vi "Analog IO.vi"() -> ()   [LabVIEW 2011]
panel:
  out "Ch9 Data 2":dbl
  out "Ch0 Data 2":dbl
  out "Ch1 Data 2":dbl
  out "Ch6 Data 2":dbl
  out "Ch2 Data 2":dbl
  out "Ch7 Data 2":dbl
  out "Ch10 Data 2":dbl
  out "Ch12 Data 2":dbl
  out "Ch13 Data 2":dbl
  out "Ch4 Data 2":dbl
  out "Ch3 Data 2":dbl
  out "Ch15 Data 2":dbl
  out "Ch14 Data 2":dbl
  out "Ch5 Data 2":dbl
  out "Ch8 Data 2":dbl
  out "Ch11 Data 2":dbl
  in  "Ch9 Range Type":i16
  in  "Ch0 Range Type":i16
  in  "Ch1 Range Type":i16
  in  "Ch6 Range Type":i16
  in  "Ch2 Range Type":i16
  in  "Ch7 Range Type":i16
  in  "Ch10 Range Type":i16
  in  "Ch12 Range Type":i16
  in  "Ch13 Range Type":i16
  in  "Ch4 Range Type":i16
  in  "Ch3 Range Type":i16
  in  "Ch15 Range Type":i16
  in  "Ch14 Range Type":i16
  in  "Ch5 Range Type":i16
  in  "Ch8 Range Type":i16
  in  "Ch11 Range Type":i16
  in  "Ch0 Data":i16
  in  "Ch15 Data":i16
  in  "Ch14 Data":i16
  in  "Ch13 Data":i16
  in  "Ch12 Data":i16
  in  "Ch11 Data":i16
  in  "Ch10 Data":i16
  in  "Ch9 Data":i16
  in  "Ch8 Data":i16
  in  "Ch7 Data":i16
  in  "Ch6 Data":i16
  in  "Ch5 Data":i16
  in  "Ch4 Data":i16
  in  "Ch3 Data":i16
  in  "Ch2 Data":i16
  in  "Ch1 Data":i16
  out "CalFault":bool
  out "Calibrating":bool
  out "AnalogGroupFault":bool
  in  "Channel Status":u32 format="%032b"
  out "Ch1Underrange":bool
  out "Ch15Underrange":bool
  out "Ch14Underrange":bool
  out "Ch13Underrange":bool
  out "Ch12Underrange":bool
  out "Ch11Underrange":bool
  out "Ch10Underrange":bool
  out "Ch9Underrange":bool
  out "Ch8Underrange":bool
  out "Ch7Underrange":bool
  out "Ch6Underrange":bool
  out "Ch5Underrange":bool
  out "Ch4Underrange":bool
  out "Ch3Underrange":bool
  out "Ch2Underrange":bool
  out "Ch0Underrange":bool
  out "Ch1Overrange":bool
  out "Ch15Overrange":bool
  out "Ch14Overrange":bool
  out "Ch13Overrange":bool
  out "Ch12Overrange":bool
  out "Ch11Overrange":bool
  out "Ch10Overrange":bool
  out "Ch9Overrange":bool
  out "Ch8Overrange":bool
  out "Ch7Overrange":bool
  out "Ch6Overrange":bool
  out "Ch5Overrange":bool
  out "Ch4Overrange":bool
  out "Ch3Overrange":bool
  out "Ch2Overrange":bool
  out "Ch0Overrange":bool
  out "Module 1":bool
  out "Module 12":bool
  out "Module 15":bool
  out "Module 14":bool
  out "Module 13":bool
  out "Module 11":bool
  out "Module 10":bool
  out "Module 9":bool
  out "Module 8":bool
  out "Module 7":bool
  out "Module 6":bool
  out "Module 5":bool
  out "Module 4":bool
  out "Module 3":bool
  out "Module 2":bool
  out "Module 0":bool
  in  "Module Faults":u16 format="%016b"
  out "Channel 1":bool
  out "Channel 15":bool
  out "Channel 14":bool
  out "Channel 13":bool
  out "Channel 12":bool
  out "Channel 11":bool
  out "Channel 10":bool
  out "Channel 9":bool
  out "Channel 8":bool
  out "Channel 7":bool
  out "Channel 6":bool
  out "Channel 5":bool
  out "Channel 4":bool
  out "Channel 3":bool
  out "Channel 2":bool
  out "Channel 0":bool
  in  "Analog Module":bool
  in  "URL":string="opc://localhost/National Instruments.NIOPCServers/ABOPC.ABEthernet.Global"
  in  "Stop Button":bool
  in  "Channel Faults":u16 format="%016b"
  # "(Volts)"
  # "Channel\nRange\nType"
  # "Channel Ranges"
  # "Channel\nFaults"
  # "Module\nFaults"
  # "Channel\nData"
  # "Under"
  # "Over"
  # "CH 0"
  # "CH 1"
  # "CH 2"
  # "CH 3"
  # "CH 4"
  # "CH 5"
  # "CH 6"
  # "CH 7"
  # "CH 8"
  # "CH 9"
  # "CH 10"
  # "CH 11"
  # "CH 12"
  # "CH 13"
  # "CH 14"
  # "CH 15"
  # "5"
  # "6"
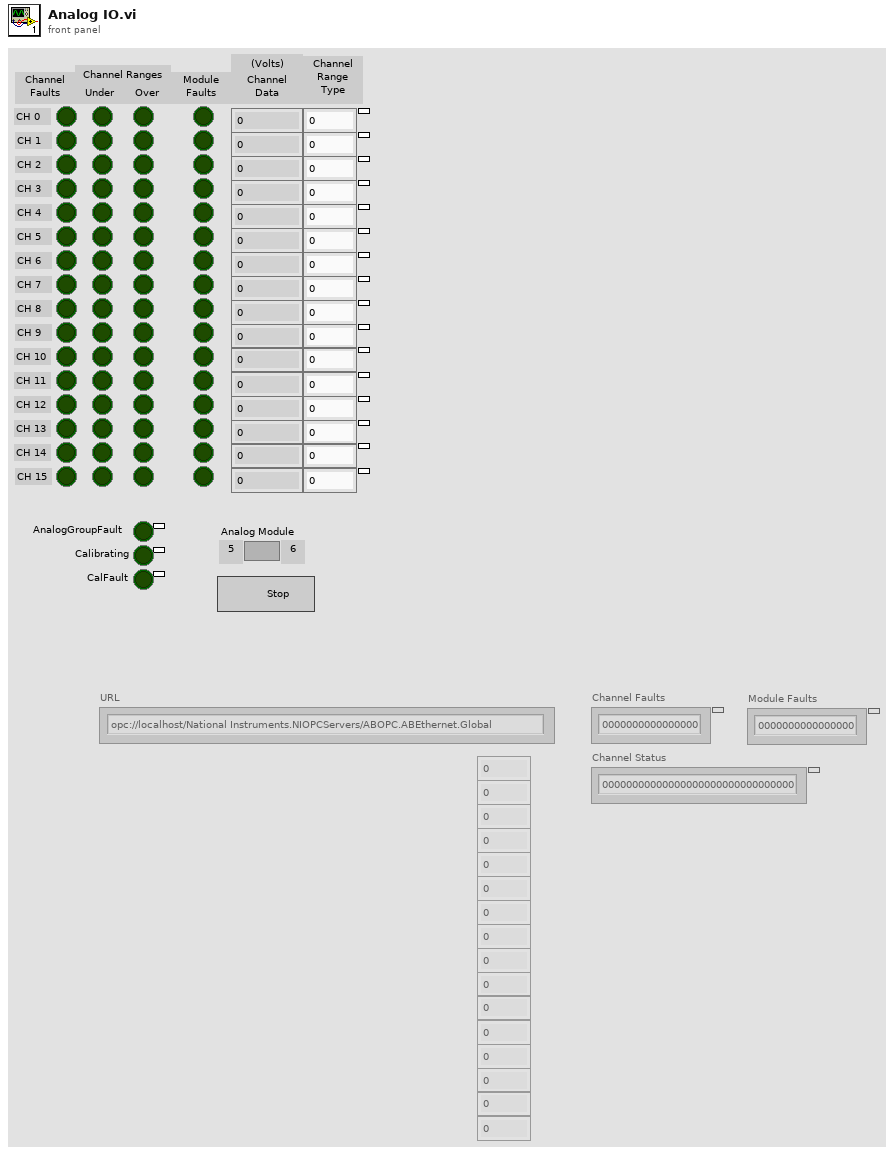
[diagram p1: front panel]
types:
  T1 = cluster{"Boolean array[0]":bool, "Boolean array[1]":bool, "Boolean array[2]":bool, "Boolean array[3]":bool, "Boolean array[4]":bool, "Boolean array[5]":bool, "Boolean array[6]":bool, "Boolean array[7]":bool, "Boolean array[8]":bool, "Boolean array[9]":bool, "Boolean array[10]":bool, "Boolean array[11]":bool, "Boolean array[12]":bool, "Boolean array[13]":bool, "Boolean array[14]":bool, "Boolean array[15]":bool}
  T2 = cluster{"[0]":dbl, "[1]":dbl, "[2]":dbl, "[3]":dbl, "[4]":dbl, "[5]":dbl, "[6]":dbl, "[7]":dbl, "[8]":dbl, "[9]":dbl, "[10]":dbl, "[11]":dbl, "[12]":dbl, "[13]":dbl, "[14]":dbl, "[15]":dbl}
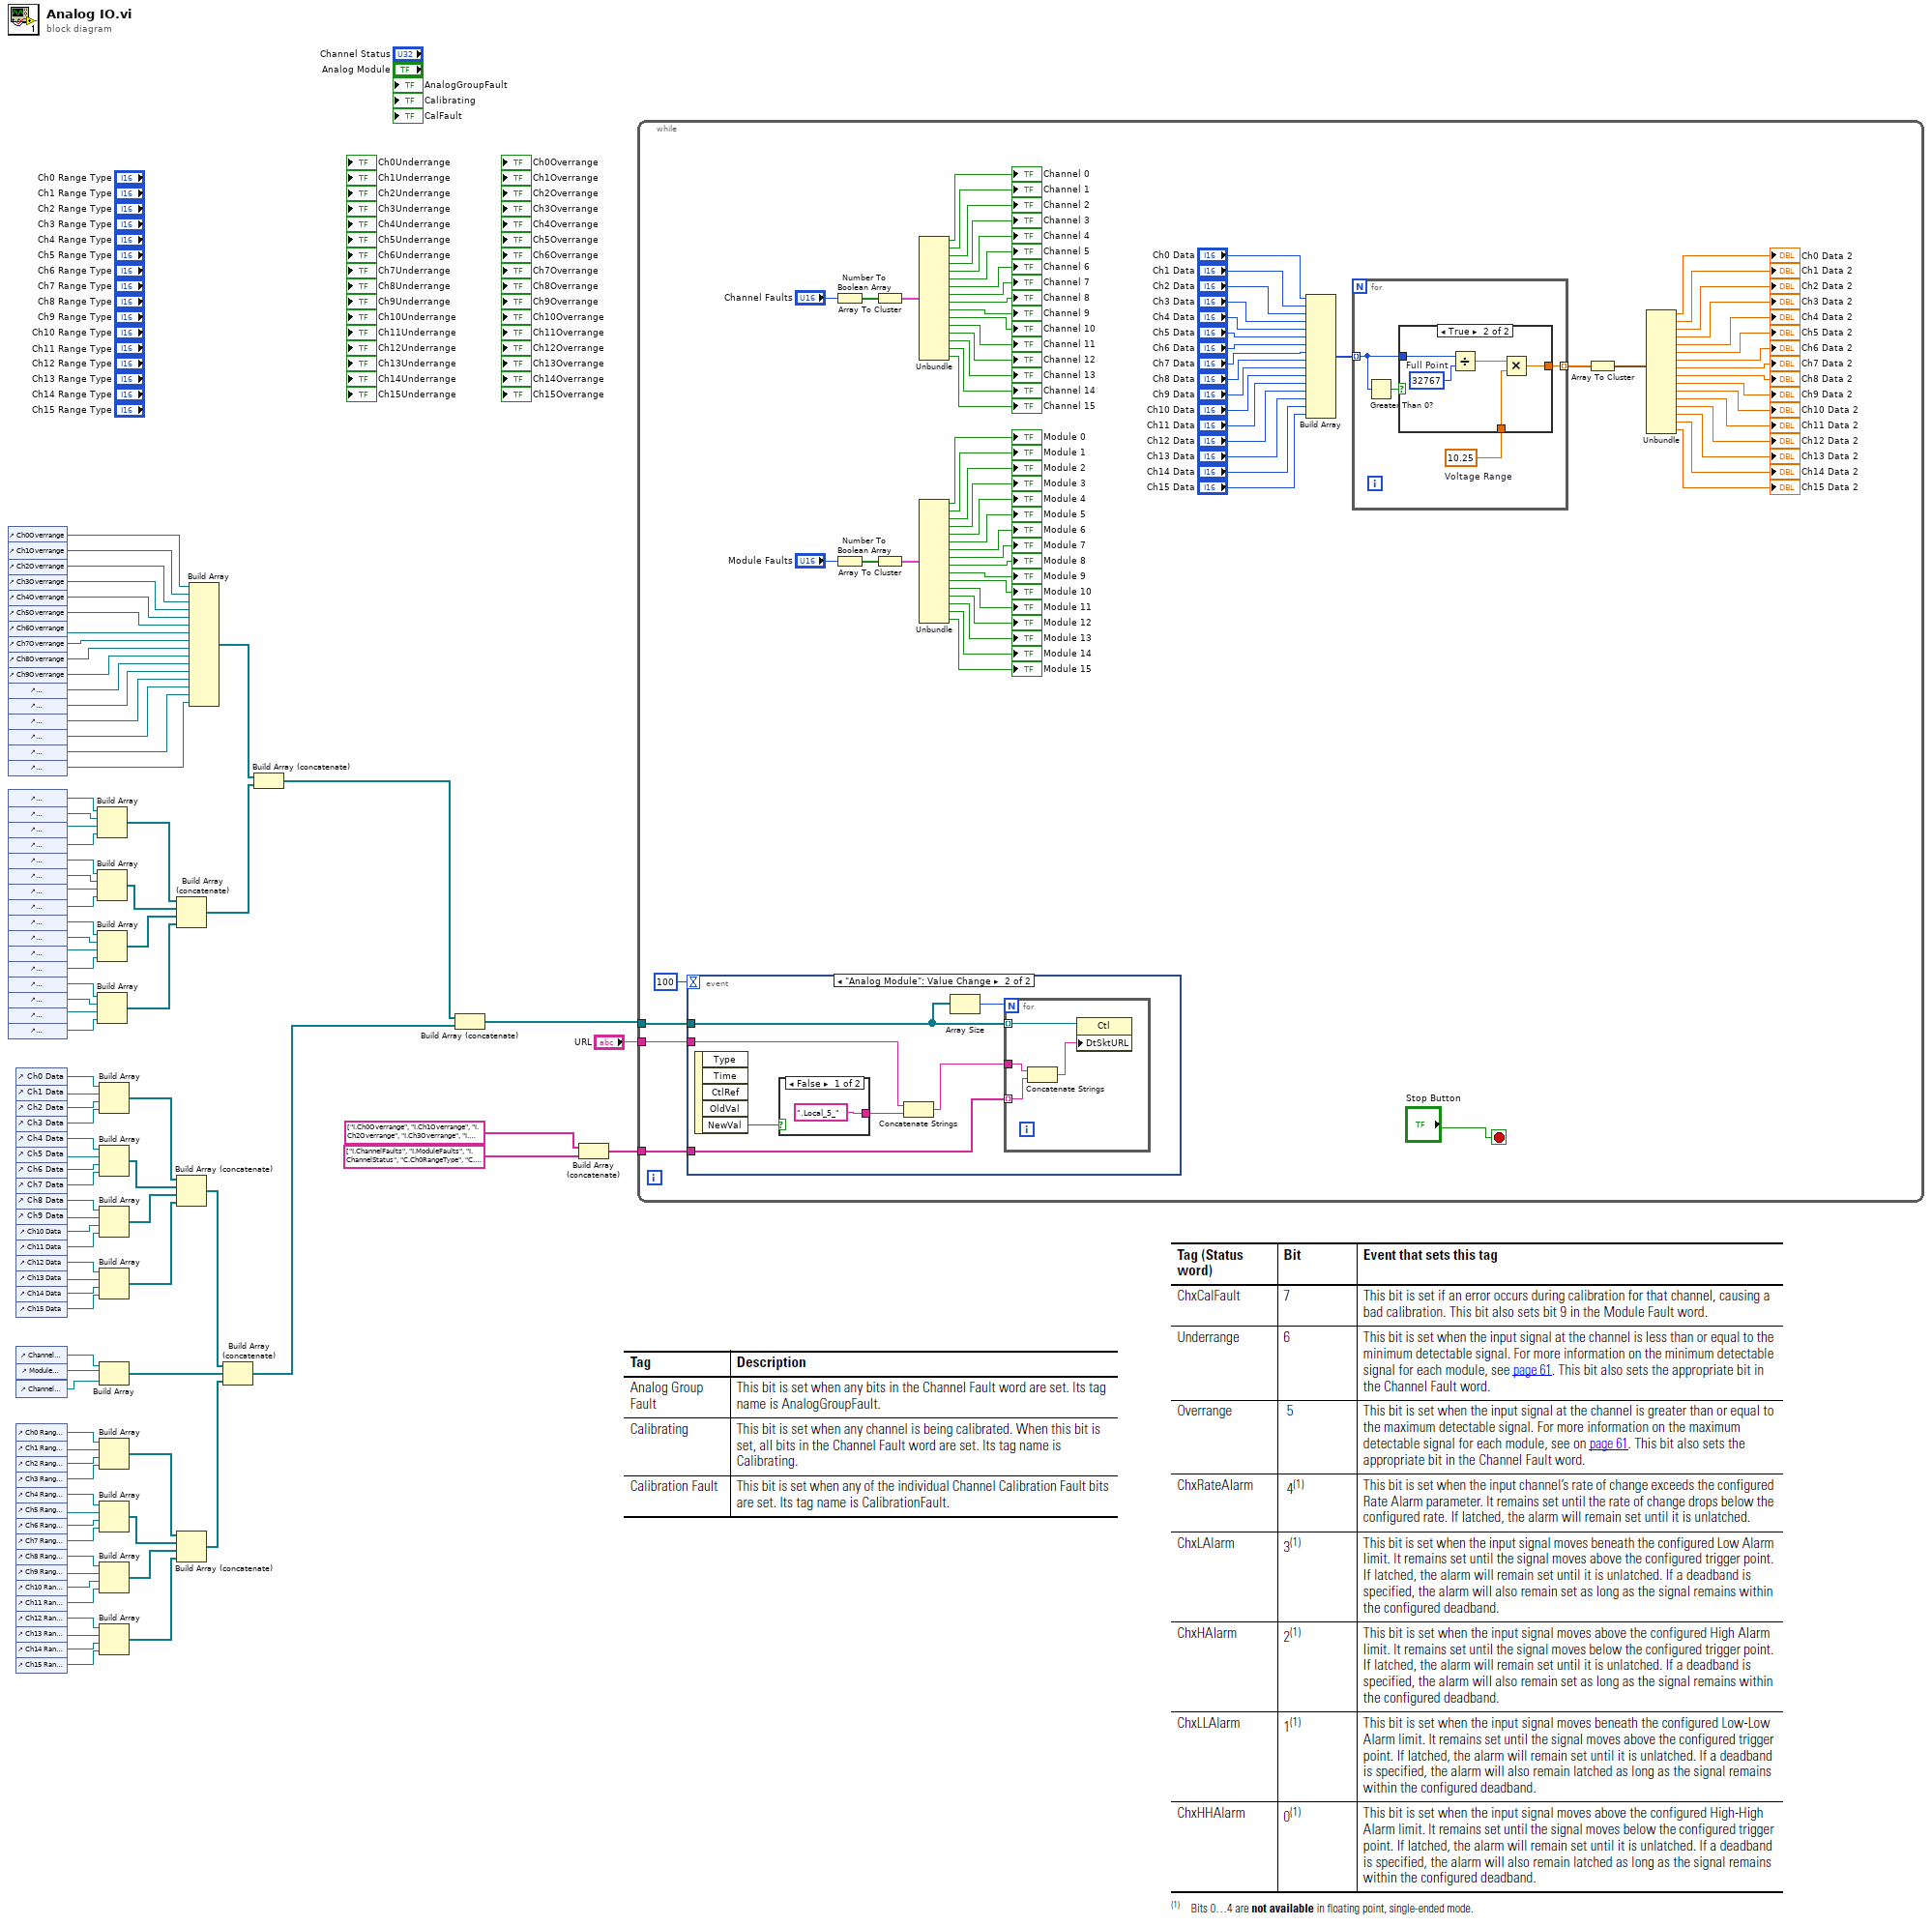
[diagram p0: block diagram]
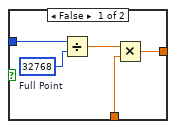
[diagram p2: hidden frame]
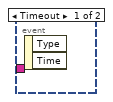
[diagram p3: hidden frame]
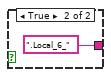
[diagram p4: hidden frame]
diagram:
  n1 = control-ref of="Ch0Overrange"() -> (w91:refnum<vi>)
  n2 = control-ref of="Ch1Overrange"() -> (w90:refnum<vi>)
  n3 = control-ref of="Ch2Overrange"() -> (w89:refnum<vi>)
  n4 = control-ref of="Ch3Overrange"() -> (w88:refnum<vi>)
  n5 = control-ref of="Ch4Overrange"() -> (w87:refnum<vi>)
  n6 = control-ref of="Ch5Overrange"() -> (w86:refnum<vi>)
  n7 = control-ref of="Ch6Overrange"() -> (w85:refnum<vi>)
  n8 = control-ref of="Ch7Overrange"() -> (w84:refnum<vi>)
  n9 = control-ref of="Ch8Overrange"() -> (w83:refnum<vi>)
  n10 = control-ref of="Ch9Overrange"() -> (w82:refnum<vi>)
  n11 = control-ref of="Ch10Overrange"() -> (w81:refnum<vi>)
  n12 = control-ref of="Ch11Overrange"() -> (w80:refnum<vi>)
  n13 = control-ref of="Ch12Overrange"() -> (w79:refnum<vi>)
  n14 = control-ref of="Ch13Overrange"() -> (w78:refnum<vi>)
  n15 = control-ref of="Ch14Overrange"() -> (w77:refnum<vi>)
  n16 = control-ref of="Ch15Overrange"() -> (w76:refnum<vi>)
  n17 = control-ref of="Ch0Underrange"() -> (w74:refnum<vi>)
  n18 = control-ref of="Ch1Underrange"() -> (w73:refnum<vi>)
  n19 = control-ref of="Ch2Underrange"() -> (w72:refnum<vi>)
  n20 = control-ref of="Ch3Underrange"() -> (w71:refnum<vi>)
  n21 = control-ref of="Ch4Underrange"() -> (w70:refnum<vi>)
  n22 = control-ref of="Ch5Underrange"() -> (w69:refnum<vi>)
  n23 = control-ref of="Ch6Underrange"() -> (w68:refnum<vi>)
  n24 = control-ref of="Ch7Underrange"() -> (w67:refnum<vi>)
  n25 = control-ref of="Ch8Underrange"() -> (w66:refnum<vi>)
  n26 = control-ref of="Ch9Underrange"() -> (w65:refnum<vi>)
  n27 = control-ref of="Ch10Underrange"() -> (w64:refnum<vi>)
  n28 = control-ref of="Ch11Underrange"() -> (w63:refnum<vi>)
  n29 = control-ref of="Ch12Underrange"() -> (w62:refnum<vi>)
  n30 = control-ref of="Ch13Underrange"() -> (w61:refnum<vi>)
  n31 = control-ref of="Ch14Underrange"() -> (w60:refnum<vi>)
  n32 = control-ref of="Ch15Underrange"() -> (w59:refnum<vi>)
  n33 = control-ref of="Ch0 Data"() -> (w50:refnum<vi>)
  n34 = control-ref of="Ch1 Data"() -> (w49:refnum<vi>)
  n35 = control-ref of="Ch2 Data"() -> (w48:refnum<vi>)
  n36 = control-ref of="Ch3 Data"() -> (w47:refnum<vi>)
  n37 = control-ref of="Ch4 Data"() -> (w46:refnum<vi>)
  n38 = control-ref of="Ch5 Data"() -> (w45:refnum<vi>)
  n39 = control-ref of="Ch6 Data"() -> (w44:refnum<vi>)
  n40 = control-ref of="Ch7 Data"() -> (w43:refnum<vi>)
  n41 = control-ref of="Ch8 Data"() -> (w42:refnum<vi>)
  n42 = control-ref of="Ch9 Data"() -> (w41:refnum<vi>)
  n43 = control-ref of="Ch10 Data"() -> (w39:refnum<vi>)
  n44 = control-ref of="Ch11 Data"() -> (w40:refnum<vi>)
  n45 = control-ref of="Ch12 Data"() -> (w38:refnum<vi>)
  n46 = control-ref of="Ch13 Data"() -> (w37:refnum<vi>)
  n47 = control-ref of="Ch14 Data"() -> (w36:refnum<vi>)
  n48 = control-ref of="Ch15 Data"() -> (w35:refnum<vi>)
  n49 = control-ref of="Channel Faults"() -> (w32:refnum<vi>)
  n50 = control-ref of="Module Faults"() -> (w33:refnum<vi>)
  n51 = control-ref of="Channel Status"() -> (w34:refnum<vi>)
  n52 = control-ref of="Ch0 Range Type"() -> (w19:refnum<vi>)
  n53 = control-ref of="Ch1 Range Type"() -> (w18:refnum<vi>)
  n54 = control-ref of="Ch2 Range Type"() -> (w17:refnum<vi>)
  n55 = control-ref of="Ch3 Range Type"() -> (w16:refnum<vi>)
  n56 = control-ref of="Ch4 Range Type"() -> (w15:refnum<vi>)
  n57 = control-ref of="Ch5 Range Type"() -> (w14:refnum<vi>)
  n58 = control-ref of="Ch6 Range Type"() -> (w13:refnum<vi>)
  n59 = control-ref of="Ch7 Range Type"() -> (w12:refnum<vi>)
  n60 = control-ref of="Ch8 Range Type"() -> (w11:refnum<vi>)
  n61 = control-ref of="Ch9 Range Type"() -> (w10:refnum<vi>)
  n62 = control-ref of="Ch10 Range Type"() -> (w8:refnum<vi>)
  n63 = control-ref of="Ch11 Range Type"() -> (w9:refnum<vi>)
  n64 = control-ref of="Ch12 Range Type"() -> (w7:refnum<vi>)
  n65 = control-ref of="Ch13 Range Type"() -> (w6:refnum<vi>)
  n66 = control-ref of="Ch14 Range Type"() -> (w5:refnum<vi>)
  n67 = control-ref of="Ch15 Range Type"() -> (w4:refnum<vi>)
  n68 = Build Array(w74, w73, w72, w71) -> (w58:refnum<vi>[])
  n69 = Build Array(w70, w69, w68, w67) -> (w57:refnum<vi>[])
  n70 = Build Array(w66, w65, w64, w63) -> (w56:refnum<vi>[])
  n71 = Build Array(w62, w61, w60, w59) -> (w55:refnum<vi>[])
  n72 = Build Array(w50, w49, w48, w47) -> (w54:refnum<vi>[])
  n73 = Build Array(w46, w45, w44, w43) -> (w53:refnum<vi>[])
  n74 = Build Array(w42, w41, w39, w40) -> (w52:refnum<vi>[])
  n75 = Build Array(w38, w37, w36, w35) -> (w51:refnum<vi>[])
  n76 = Build Array(w32, w33, w34) -> (w2:refnum<vi>[])
  n77 = Build Array(w19, w18, w17, w16) -> (w23:refnum<vi>[])
  n78 = Build Array(w15, w14, w13, w12) -> (w22:refnum<vi>[])
  n79 = Build Array(w11, w10, w8, w9) -> (w21:refnum<vi>[])
  n80 = Build Array(w7, w6, w5, w4) -> (w20:refnum<vi>[])
  n81 = Build Array (concatenate)(w58, w57, w56, w55) -> (w30:refnum<vi>[])
  n82 = Build Array (concatenate)(w54, w53, w52, w51) -> (w3:refnum<vi>[])
  n83 = Build Array (concatenate)(w23, w22, w21, w20) -> (w1:refnum<vi>[])
  n84 = Build Array(w91, w90, w89, w88, w87, w86, w85, w84, w83, w82, w81, w80, w79, w78, w77, w76) -> (w31:refnum<vi>[])
  n85 = Build Array (concatenate)(w3, w2, w1) -> (w27:refnum<vi>[])
  n86 = Build Array (concatenate)(w31, w30) -> (w28:refnum<vi>[])
  n87 = Build Array (concatenate)(w28, w27) -> (w29:refnum<vi>[])
  n88 = Build Array (concatenate)(string[] ["I.Ch0Overrange", "I.Ch1Overrange", "I.Ch2Overrange", "I.Ch3Overrange", "I.Ch4Overrange", "I.Ch5Overrange", "I.Ch6Overrange", "I.Ch7Overrange", "I.Ch8Overrange", "I.Ch9Overrange", "I.Ch10Overrange", "I.Ch11Overrange", "I.Ch12Overrange", "I.Ch13Overrange", "I.Ch14Overrange", "I.Ch15Overrange", "I.Ch0Underrange", "I.Ch1Underrange", "I.Ch2Underrange", "I.Ch3Underrange", "I.Ch4Underrange", "I.Ch5Underrange", "I.Ch6Underrange", "I.Ch7Underrange", "I.Ch8Underrange", "I.Ch9Underrange", "I.Ch10Underrange", "I.Ch11Underrange", "I.Ch12Underrange", "I.Ch13Underrange", "I.Ch14Underrange", "I.Ch15Underrange", "I.Ch0Data", "I.Ch1Data", "I.Ch2Data", "I.Ch3Data", "I.Ch4Data", "I.Ch5Data", "I.Ch6Data", "I.Ch7Data", "I.Ch8Data", "I.Ch9Data", "I.Ch10Data", "I.Ch11Data", "I.Ch12Data", "I.Ch13Data", "I.Ch14Data", "I.Ch15Data"], string[] ["I.ChannelFaults", "I.ModuleFaults", "I.ChannelStatus", "C.Ch0RangeType", "C.Ch1RangeType", "C.Ch2RangeType", "C.Ch3RangeType", "C.Ch4RangeType", "C.Ch5RangeType", "C.Ch6RangeType", "C.Ch7RangeType", "C.Ch8RangeType", "C.Ch9RangeType", "C.Ch10RangeType", "C.Ch11RangeType", "C.Ch12RangeType", "C.Ch13RangeType", "C.Ch14RangeType", "C.Ch15RangeType"]) -> (w24:string[])
  n89 = while {
    tunnel: "URL" -> [w167]
    tunnel: w24 -> [w128]
    tunnel: w29 -> [w127]
    stop <- "Stop Button" stop-if-true
    n90 = event shown="[1] \"Analog Module\": Value Change" {
      selector: _ -> [_ _]
      dyn-events: _ -> [_ _]
      timeout: 100 -> [_ _]
      tunnel: w167 -> [_ w187]
      tunnel: w128 -> [_ w189]
      tunnel: w127 -> [_ w184]
      event Timeout {
        n91 = event-data() -> ()  [unwired: 1 in, 2 out]
      }
      event "Analog Module": Value Change {
        n92 = event-data() -> ("NewVal"=w190:bool)  [unwired: 1 in, 4 out]
        n93 = case shown="False" w190 {
          tunnel: [".Local_5_" ".Local_6_"] -> w188
          frame False {
          }
          frame True {
          }
        }
        n94 = Concatenate Strings(w187, w188) -> (w186:string)
        n95 = Array Size(array=w184) -> (size(s)=w185:i32)
        n96 = for {
          N: w185 -> [_]
          tunnel: w189 -> [w194] mode=indexing
          tunnel: w184 -> [w191] mode=indexing
          tunnel: w186 -> [w192]
          n97 = Concatenate Strings(w192, w194) -> (w193:string)
          n98 = property on="Property Node" class="Ctl"(reference=w191, "DtSktURL"=w193) -> ()  [unwired: 1 in, 2 out]
        }
      }
    }
    n99 = Number To Boolean Array(number="Channel Faults") -> (Boolean array=w165:bool[])
    n100 = Number To Boolean Array(number="Module Faults") -> (Boolean array=w147:bool[])
    n101 = Array To Cluster(array=w165) -> (cluster=w164:T1)
    n102 = Array To Cluster(array=w147) -> (cluster=w146:T1)
    n103 = Unbundle(w164) -> ("Boolean array[0]"=→"Channel 0":bool, "Boolean array[1]"=→"Channel 1":bool, "Boolean array[2]"=→"Channel 2":bool, "Boolean array[3]"=→"Channel 3":bool, "Boolean array[4]"=→"Channel 4":bool, "Boolean array[5]"=→"Channel 5":bool, "Boolean array[6]"=→"Channel 6":bool, "Boolean array[7]"=→"Channel 7":bool, "Boolean array[8]"=→"Channel 8":bool, "Boolean array[9]"=→"Channel 9":bool, "Boolean array[10]"=→"Channel 10":bool, "Boolean array[11]"=→"Channel 11":bool, "Boolean array[12]"=→"Channel 12":bool, "Boolean array[13]"=→"Channel 13":bool, "Boolean array[14]"=→"Channel 14":bool, "Boolean array[15]"=→"Channel 15":bool)
    n104 = Unbundle(w146) -> ("Boolean array[0]"=→"Module 0":bool, "Boolean array[1]"=→"Module 1":bool, "Boolean array[2]"=→"Module 2":bool, "Boolean array[3]"=→"Module 3":bool, "Boolean array[4]"=→"Module 4":bool, "Boolean array[5]"=→"Module 5":bool, "Boolean array[6]"=→"Module 6":bool, "Boolean array[7]"=→"Module 7":bool, "Boolean array[8]"=→"Module 8":bool, "Boolean array[9]"=→"Module 9":bool, "Boolean array[10]"=→"Module 10":bool, "Boolean array[11]"=→"Module 11":bool, "Boolean array[12]"=→"Module 12":bool, "Boolean array[13]"=→"Module 13":bool, "Boolean array[14]"=→"Module 14":bool, "Boolean array[15]"=→"Module 15":bool)
    n105 = Build Array("Ch0 Data", "Ch1 Data", "Ch2 Data", "Ch3 Data", "Ch4 Data", "Ch5 Data", "Ch6 Data", "Ch7 Data", "Ch8 Data", "Ch9 Data", "Ch10 Data", "Ch11 Data", "Ch12 Data", "Ch13 Data", "Ch14 Data", "Ch15 Data") -> (w110:i16[])
    n106 = for {
      tunnel: w110 -> [w172] mode=indexing
      tunnel: [w173] -> w109 mode=indexing
      w170 = 10.25  # Voltage Range
      n107 = Greater Than 0?(x=w172) -> (x > 0?=w171:bool)
      n108 = case shown="True" w171 {
        tunnel: w172 -> [w175 w183]
        tunnel: [w174 w181] -> w173
        tunnel: w170 -> [w176 w180]
        frame False {
          w177 = 32768  # Full Point
          n109 = Divide(x=w175, y=w177) -> (x/y=w178:dbl)
          n110 = Multiply(x=w178, y=w176) -> (x*y=w174:dbl)
        }
        frame True {
          w179 = 32767  # Full Point
          n111 = Divide(x=w183, y=w179) -> (x/y=w182:dbl)
          n112 = Multiply(x=w182, y=w180) -> (x*y=w181:dbl)
        }
      }
    }
    n113 = Array To Cluster(array=w109) -> (cluster=w108:T2)
    n114 = Unbundle(w108) -> ("[0]"=→"Ch0 Data 2":dbl, "[1]"=→"Ch1 Data 2":dbl, "[2]"=→"Ch2 Data 2":dbl, "[3]"=→"Ch3 Data 2":dbl, "[4]"=→"Ch4 Data 2":dbl, "[5]"=→"Ch5 Data 2":dbl, "[6]"=→"Ch6 Data 2":dbl, "[7]"=→"Ch7 Data 2":dbl, "[8]"=→"Ch8 Data 2":dbl, "[9]"=→"Ch9 Data 2":dbl, "[10]"=→"Ch10 Data 2":dbl, "[11]"=→"Ch11 Data 2":dbl, "[12]"=→"Ch12 Data 2":dbl, "[13]"=→"Ch13 Data 2":dbl, "[14]"=→"Ch14 Data 2":dbl, "[15]"=→"Ch15 Data 2":dbl)
  }
